vi "S2DS_Generate 2D data.vi"(7 "2D data in":dbl[][](array[numeric]), 8 "1D data in":dbl[](array[numeric]), 9 "Factors":dbl[](array[numeric])) -> (2 "2D data out":dbl[][](array[numeric]))   [LabVIEW 2025]
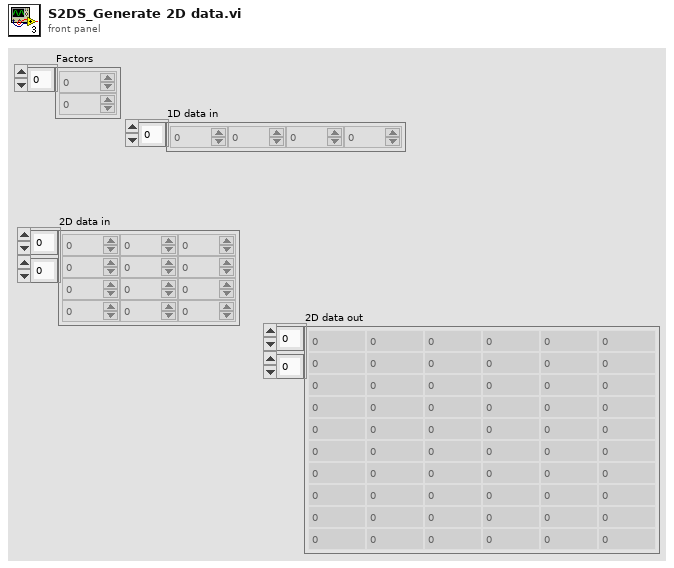
[diagram p1: front panel]
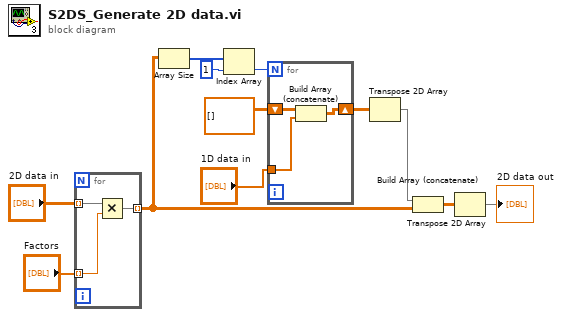
[diagram p0: block diagram]
diagram:
  n1 = for {
    tunnel: "Factors" -> [w14] mode=indexing
    tunnel: "2D data in" -> [w15] mode=indexing
    tunnel: [w13] -> w2 mode=indexing
    n2 = Multiply(x=w15, y=w14) -> (x*y=w13:dbl[])
  }
  n3 = Array Size(array=w2) -> (size(s)=w12:i32[])
  n4 = Index Array(array=w12, index=1) -> (element=w4:i32)
  n5 = for {
    N: w4 -> [_]
    tunnel: "1D data in" -> [w18]
    shift-right: [w17] -> w9
    shift-left: dbl[][] [] -> [w16]
    n6 = Build Array (concatenate)(w16, w18) -> (w17:dbl[][])
  }
  n7 = Transpose 2D Array(2D array=w9) -> (transposed array=w8:dbl[][])
  n8 = Build Array (concatenate)(w8, w2) -> (w7:dbl[][])
  n9 = Transpose 2D Array(2D array=w7) -> (transposed array=→"2D data out":dbl[][])
